vi "多反-镜像-缺陷检测.vi"(4 "底线中心到头部中心偏移量参数":dbl=100.0 format="%#_13g", 5 "头部拟合直径参数":dbl=110.0 format="%#_13g", 7 "胶木铜碎面具偏移_右上0起逆时针":sgl[](array[numeric])=[190.0, 190.0, 190.0, 190.0, 190.0, 190.0, 190.0, 190.0, 190.0, 190.0], 8 "ImgTmps":T8(array[cluster]), 9 "白条面积限度":dbl=200.0 format="%#_13g", 10 "多反调用参数":T9={"IMG_FULL_GRAY_HEAD"=refnum, "IMG_SRC_RO"=refnum, "IMG_Prod_Body_RO"=refnum, "Size_Msk_Half"=0.0, "ROI_Cent"={"Global Rectangle"=[], "Contours"=[]}, "ROI_Prod_Raw"={"Global Rectangle"=[], "Contours"=[]}, "SlotAngles"=[], "img_H_copSlices"=[], "MirroredAngle"=0.0, "SlotCopperParams"={"向外延伸距离"=65.0, "向内延伸距离"=42.0, "排除间隔"=3.0}, "ROIs_Prod_Raw"=[], "MirroredAngles"=[]} {"ROIs_Prod_Raw"."Contours"."Type" items=["No Selection", "Point", "Line", "Rectangle", "Oval", "Polygon", "Freehand Region", "Annulus", "Unused2", "Unused3", "Broken Line", "Freehand Line", "Rotated Rectangle"]; "ROI_Cent"."Contours"."Type" items=["No Selection", "Point", "Line", "Rectangle", "Oval", "Polygon", "Freehand Region", "Annulus", "Unused2", "Unused3", "Broken Line", "Freehand Line", "Rotated Rectangle"]; "ROI_Prod_Raw"."Contours"."Type" items=["No Selection", "Point", "Line", "Rectangle", "Oval", "Polygon", "Freehand Region", "Annulus", "Unused2", "Unused3", "Broken Line", "Freehand Line", "Rotated Rectangle"]}, 11 "镜像编号":i32) -> (0 "ms":cluster{u32, u32, u32}, 1 "头缺量":dbl, 2 "输出簇":T4 {"ROI头缺检测显示"."Contours"."Type" items=["No Selection", "Point", "Line", "Rectangle", "Oval", "Polygon", "Freehand Region", "Annulus", "Unused2", "Unused3", "Broken Line", "Freehand Line", "Rotated Rectangle"]}, 3 "Image Dst Out":T2, 6 "钩外多胶正常":bool)   [LabVIEW 2018]
uses:
  <vilib>/vision/Image Controls.llb/IMAQ Image.ctl
  <vilib>/vision/Measure.llb/Edge Options.ctl
  <vilib>/vision/Measure.llb/Edge Polarity.ctl
  <vilib>/vision/NI_Vision_Development_Module.lvlib
panel:
  in  "原始模板尺寸":T1={"Left"=0, "Top"=0, "Right"=700, "Bottom"=700, "Rotation"=0.0} {"Rotation" format="%.2f"; "Left" scale=0.0..1024.0; "Right" scale=0.0..1024.0}
  out "Image 3":T2(plugin-control)
  out "脏污检测图像":T2(plugin-control)
  out "脏污所处位置信息":dbl[][](array[numeric]) format="%.2f"
  out "脏污数量":i32
  in  "脏污面积下限":T5(array[cluster])=[{"Measurement Parameter"=35, "Range Lower Value"=0.0, "Range Upper Value"=1000.0, "Range"=FALSE, "Measurement Type"=FALSE}] {"Measurement Parameter" items=["Center of Mass X", "Center of Mass Y", "First Pixel X", "First Pixel Y", "Bounding Rect Left", "Bounding Rect Top", "Bounding Rect Right", "Bounding Rect Bottom", "Max Feret Diameter Start X", "Max Feret Diameter Start Y", "Max Feret Diameter End X", "Max Feret Diameter End Y", "Max Horiz. Segment Length Left", "Max Horiz. Segment Length Right", "Max Horiz. Segment Length Row", "-", "Bounding Rect Width", "Bounding Rect Height", "Bounding Rect Diagonal", "Perimeter", "Convex Hull Perimeter", "Holes' Perimeter", "Max Feret Diameter", "Equivalent Ellipse Major Axis", "Equivalent Ellipse Minor Axis", "Equivalent Ellipse Minor Axis (Feret)", "Equivalent Rect Long Side", "Equivalent Rect Short Side", "Equivalent Rect Diagonal", "Equivalent Rect Short Side (Feret)", "Average Horiz. Segment Length", "Average Vert. Segment Length", "Hydraulic Radius", "Waddel Disk Diameter", "-", "Area", "Holes' Area", "Particle & Holes' Area", "Convex Hull Area", "Image Area", "-", "Number of Holes", "Number of Horiz. Segments", "Number of Vert. Segments", "-", "Orientation", "Max Feret Diameter Orientation", "-", "% Area/Image Area", "% Area/(Particle & Holes' Area)", "Ratio of Equivalent Ellipse Axes", "Ratio of Equivalent Rect Sides", "-", "Elongation Factor", "Compactness Factor", "Heywood Circularity Factor", "Type Factor", "-", "Sum X", "Sum Y", "Sum XX", "Sum XY", "Sum YY", "Sum XXX", "Sum XXY", "Sum XYY", "Sum YYY", "-", "Moment of Inertia XX", "Moment of Inertia XY", "Moment of Inertia YY", "Moment of Inertia XXX", "Moment of Inertia XXY", "Moment of Inertia XYY", "Moment of Inertia YYY", "Norm. Moment of Inertia XX", "Norm. Moment of Inertia XY", "Norm. Moment of Inertia YY", "Norm. Moment of Inertia XXX", "Norm. Moment of Inertia XXY", "Norm. Moment of Inertia XYY", "Norm. Moment of Inertia YYY", "Hu Moment 1", "Hu Moment 2", "Hu Moment 3", "Hu Moment 4", "Hu Moment 5", "Hu Moment 6", "Hu Moment 7"]}
  in  "脏污灰度上限":cluster{"Lower value":sgl, "Upper value":sgl}={"Lower value"=2.0, "Upper value"=48.0}
  out "用于打探针查看":T2
  in  "检刀纹_EdgeOptions":T6={"Edge Polarity"=2, "Kernel Size"=3, "Width"=15, "Minimum Edge Strength"=50.0, "Interpolation Type"=enum."Bilinear Fixed", "Data Processing Method"=enum."Average"} {"Edge Polarity" items=["All Edges", "Rising Edges", "Falling Edges"]; "Minimum Edge Strength" format="%.2f"; "Width" step=2; "Kernel Size" step=2}
  out "中心到产品指向角":dbl
  out "Image":T2(plugin-control)
  in  "镜像编号 2":i32
  out "错误输出":errorcluster
  in  "开启调试模式":bool
  in  "开启铜碎调试显示":bool=TRUE
  in  "槽形状参数配置-槽边白条":cluster{"槽形态半长":sgl, "槽形态半宽":sgl}={"槽形态半长"=999.0, "槽形态半宽"=999.0}
  in  "Annulus":T10={"Center X"=0, "Center Y"=0, "Inner Radius"=27, "Outer Radius"=107, "Start Angle"=0.0, "End Angle"=0.0} {"End Angle" min=-90.0 max=90.0 step=1.0 format="%.2f"; "Start Angle" min=-90.0 max=90.0 step=1.0 format="%.2f"; "Center X" scale=0.0..1024.0}
  in  "钩子圆面具偏移":sgl=110.0
  in  "产品高度参考值":sgl=1.0 format="%_3g"
  out "error out 4":errorcluster
  in  "镀锡部分面具偏移_右上0起逆时针":sgl[](array[numeric])=[80.0, 80.0, 80.0, 80.0, 80.0, 80.0, 80.0, 80.0, 80.0, 80.0]
  in  "调整下限消除头部黑区稍亮部位误判作铜碎情况":cluster{"Lower value":i32, "Upper value":i32}={"Lower value"=20, "Upper value"=255}
  in  "头部缺损最大偏差":dbl=2.9999999999999982
  in  "头部边线拟合范围半角":dbl=21.0
  out "error out 6":errorcluster
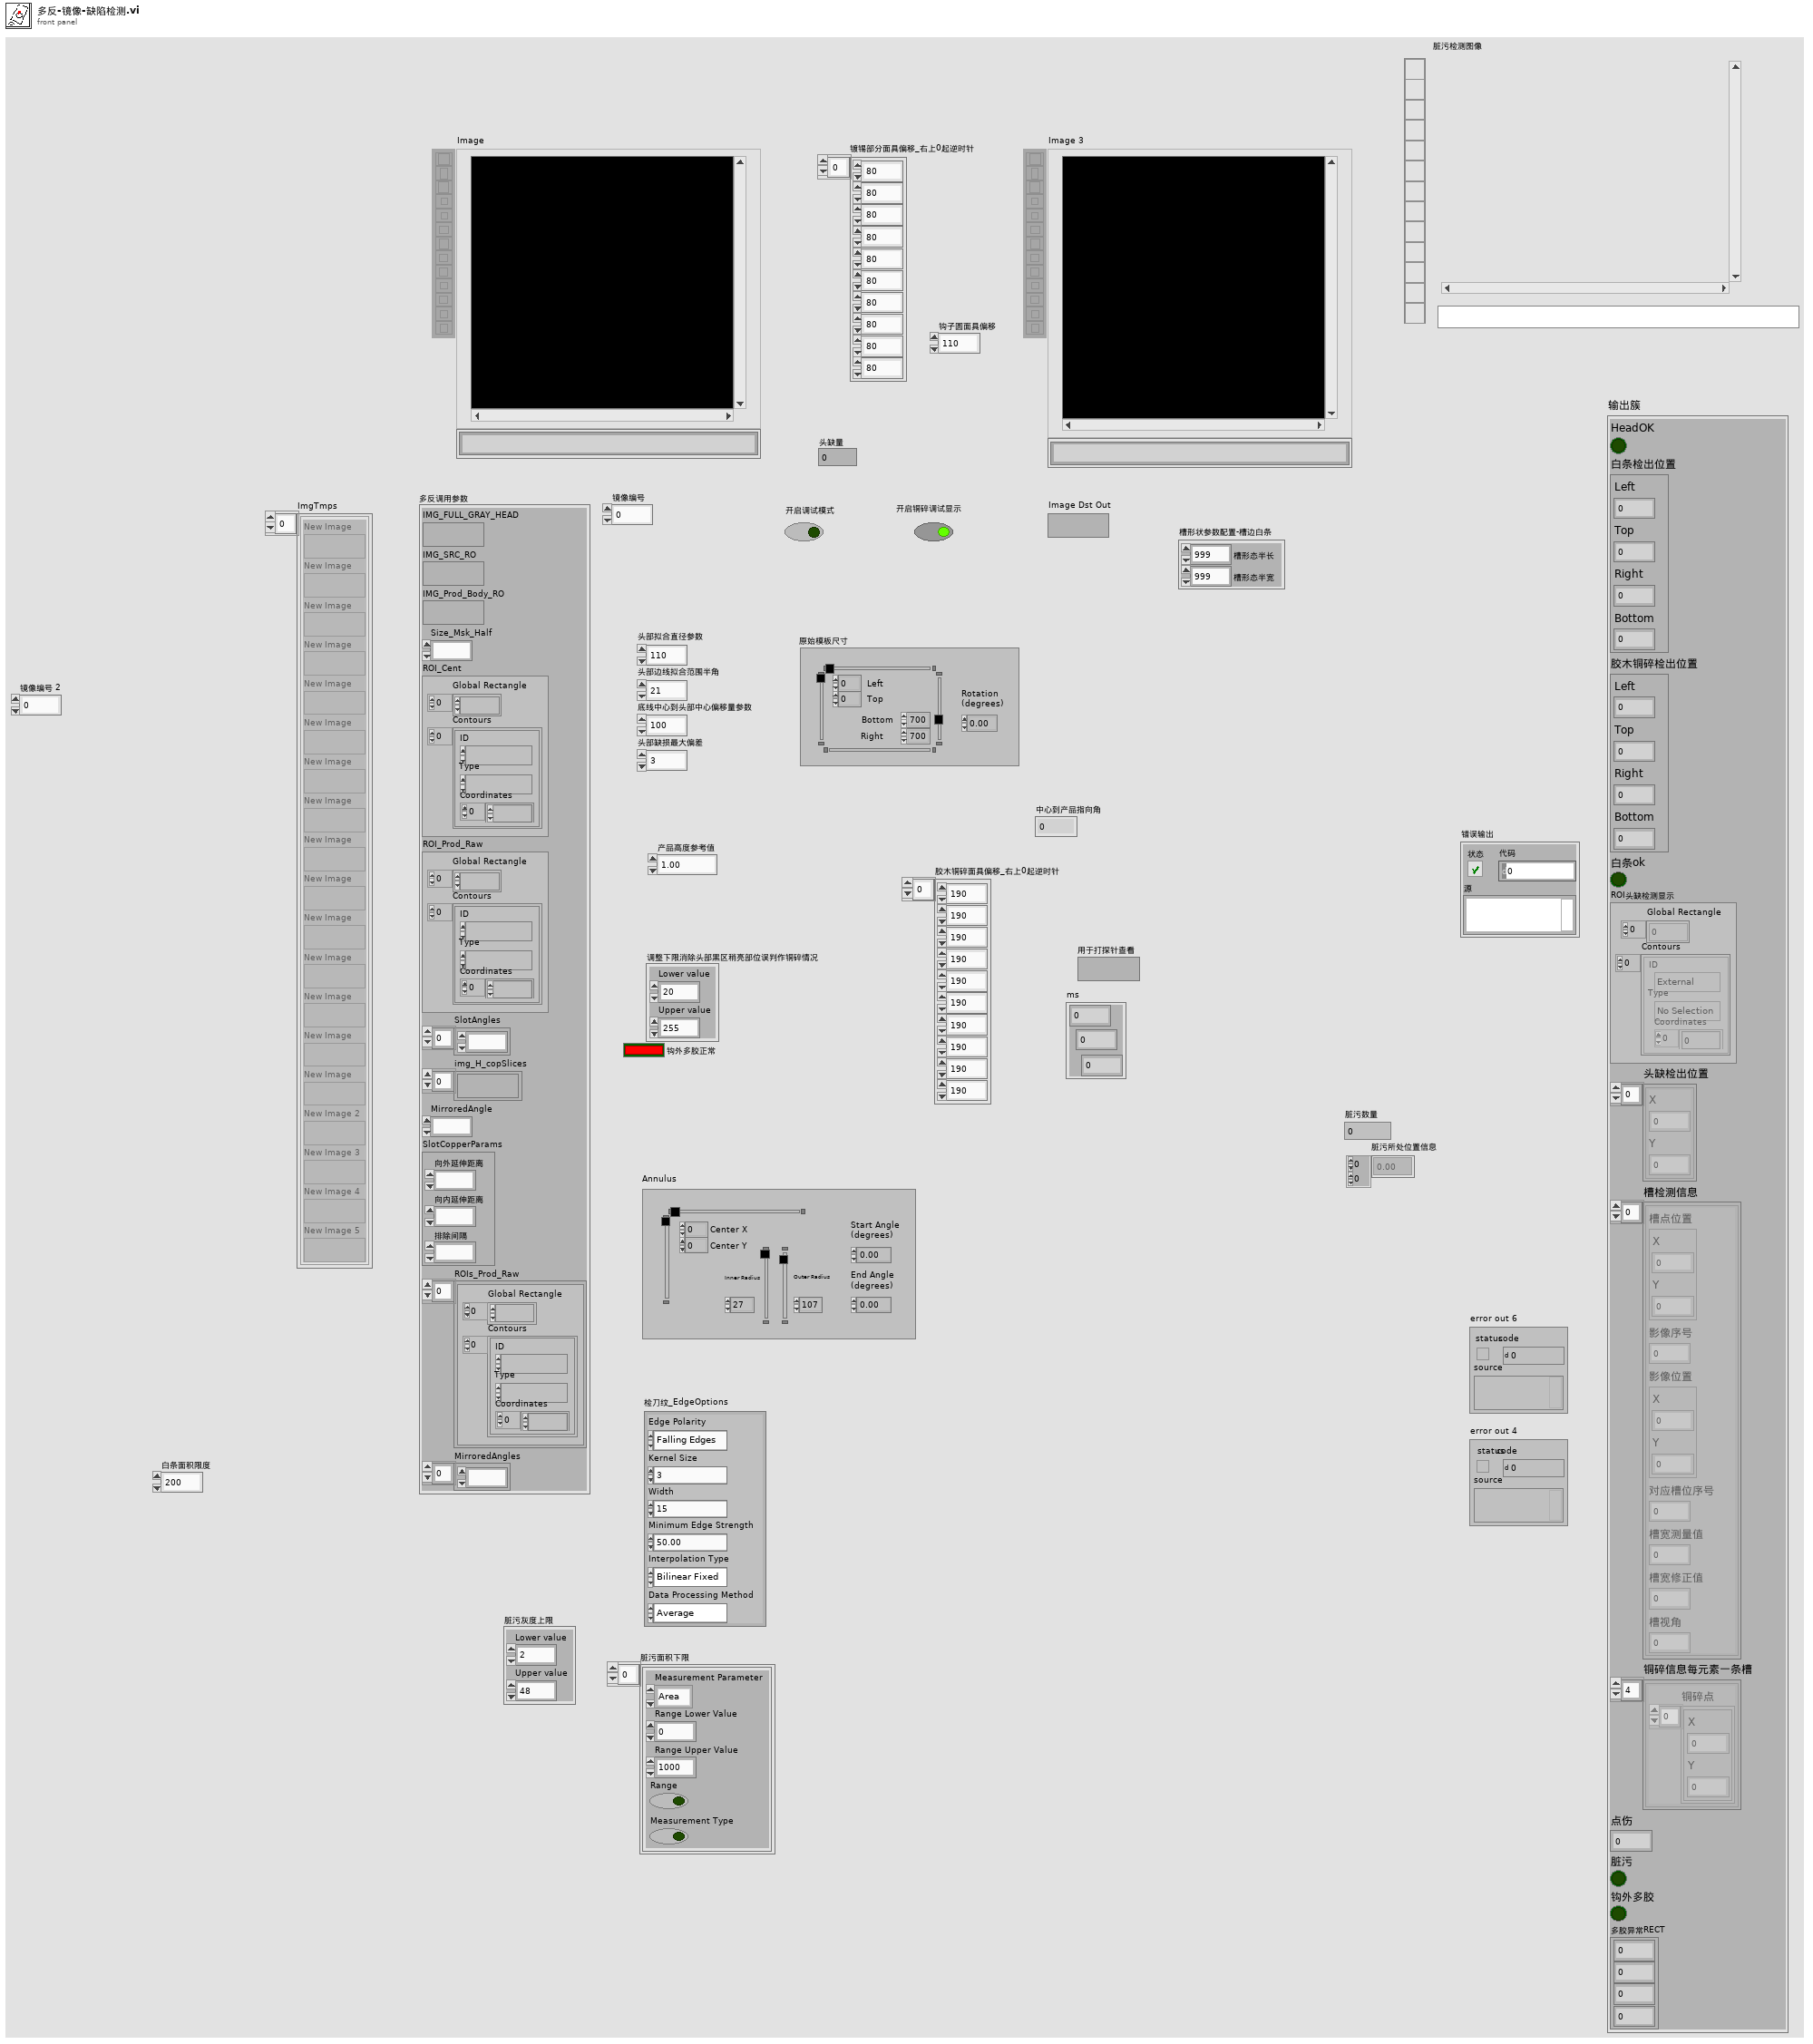
[diagram p1: front panel]
types:
  T1 = typedef "IMAQ Rectangle" = cluster{"Left":i32, "Top":i32, "Right":i32, "Bottom":i32, "Rotation":dbl}
  T2 = typedef "IMAQ Image.ctl" = refnum<image>
  T3 = typedef "ROI Descriptor" = cluster{"Global Rectangle":i32[], "Contours":cluster{"ID":enum32{"External", "Internal"}, "Type":u32, "Coordinates":i32[]}[]}
  T4 = cluster{"HeadOK":bool, "白条检出位置":cluster{"Left":i32, "Top":i32, "Right":i32, "Bottom":i32}, "胶木铜碎检出位置":cluster{"Left":i32, "Top":i32, "Right":i32, "Bottom":i32}, "白条ok":bool, "ROI头缺检测显示":T3, "头缺检出位置":cluster{"X":dbl, "Y":dbl}[], "槽检测信息":cluster{"槽点位置":cluster{"X":sgl, "Y":sgl}, "影像序号":i32, "影像位置":cluster{"X":sgl, "Y":sgl}, "对应槽位序号":i32, "槽宽测量值":dbl, "槽宽修正值":dbl, "槽视角":dbl}[], "铜碎信息每元素一条槽":cluster{"铜碎点":cluster{"X":sgl, "Y":sgl}[]}[], "点伤":dbl, "脏污":bool, "钩外多胶":bool, "多胶异常RECT":cluster{dbl, dbl, dbl, dbl}}
  T5 = cluster{"Measurement Parameter":i32, "Range Lower Value":dbl, "Range Upper Value":dbl, "Range":bool, "Measurement Type":bool}[]
  T6 = typedef "Edge Options.ctl" = cluster{"Edge Polarity":T7, "Kernel Size":u32, "Width":u32, "Minimum Edge Strength":sgl, "Interpolation Type":enum32{"Zero Order", "Bilinear", "Quadratic", "Cubic", "Bilinear Fixed"}, "Data Processing Method":enum32{"Average", "Median"}}
  T7 = typedef "Edge Polarity.ctl" = u32
  T8 = cluster{"New Image":T2, "New Image":T2, "New Image":T2, "New Image":T2, "New Image":T2, "New Image":T2, "New Image":T2, "New Image":T2, "New Image":T2, "New Image":T2, "New Image":T2, "New Image":T2, "New Image":T2, "New Image":T2, "New Image":T2, "New Image 2":T2, "New Image 3":T2, "New Image 4":T2, "New Image 5":T2}[]
  T9 = cluster{"IMG_FULL_GRAY_HEAD":T2, "IMG_SRC_RO":T2, "IMG_Prod_Body_RO":T2, "Size_Msk_Half":dbl, "ROI_Cent":T3, "ROI_Prod_Raw":T3, "SlotAngles":dbl[], "img_H_copSlices":T2[], "MirroredAngle":dbl, "SlotCopperParams":cluster{"向外延伸距离":sgl, "向内延伸距离":sgl, "排除间隔":sgl}, "ROIs_Prod_Raw":T3[], "MirroredAngles":dbl[]}
  T10 = typedef "IMAQ Circle" = cluster{"Center X":i32, "Center Y":i32, "Inner Radius":i32, "Outer Radius":i32, "Start Angle":dbl, "End Angle":dbl}
  T11 = typedef "Image Type" = u32
  T12 = enum32{"AutoM", "Close", "Dilate", "Erode", "Gradient", "Gradient out", "Gradient in", "Hit miss", "Open", "PClose", "POpen", "Thick", "Thin"}
  T13 = enum16{"Get First Edge", "Get First + Last Edge", "Get All Edges", "Get Best Edge"}
  T14 = cluster{"槽点位置":cluster{"X":sgl, "Y":sgl}, "影像序号":i32, "影像位置":cluster{"X":sgl, "Y":sgl}, "对应槽位序号":i32, "槽宽测量值":dbl, "槽宽修正值":dbl, "槽视角":dbl}[]
  T15 = cluster{"New Image":T2, "New Image":T2, "New Image":T2, "New Image":T2, "New Image":T2, "New Image":T2, "New Image":T2, "New Image":T2, "New Image":T2, "New Image":T2, "New Image":T2, "New Image":T2, "New Image":T2, "New Image":T2, "New Image":T2, "New Image 2":T2, "New Image 3":T2, "New Image 4":T2, "New Image 5":T2}
  T16 = cluster{"New Image":T2, "New Image":T2, "New Image":T2, "New Image":T2, "New Image":T2}
  T17 = cluster{"Center (Pixels)":cluster{"X":sgl, "Y":sgl}, "Radius (Pixels)":dbl, "Center (Real-World)":cluster{"X":sgl, "Y":sgl}, "Radius (Real-World)":dbl, "Roundness (Real-World)":dbl, "Average Strength":dbl, "Average SNR (dB)":dbl}
  T18 = typedef "Edge New.ctl" = cluster{"Location (Pixel)":cluster{"X":sgl, "Y":sgl}, "Location (Real-World)":cluster{"X":sgl, "Y":sgl}, "Distance (Pixel)":dbl, "Distance (Real-World)":dbl, "Strength":dbl, "Noise":dbl, "Rising?":bool}
  T19 = cluster{"width":sgl, "point":cluster{"X":sgl, "Y":sgl}}[]
  T20 = cluster{"槽点位":cluster{"X":sgl, "Y":sgl}, "产品位":cluster{"X":sgl, "Y":sgl}, "各槽角":dbl[], "中心位":cluster{"X":sgl, "Y":sgl}, "中心产品半径":sgl, "最接近槽角序号":i32, "槽在中心到产品连线所在侧":enum16{"左侧-逆时针向", "右侧-顺时针向"}, "中心位到产品位指向角":sgl}
  T21 = cluster{"产品位":cluster{"X":sgl, "Y":sgl}, "槽点位":cluster{"X":sgl, "Y":sgl}, "产品位指向角度":sgl, "产品底线半径":sgl, "向外延伸距离":sgl, "向内延伸距离":sgl, "排除间隔":sgl}
  T22 = cluster{"槽点位置":cluster{"X":sgl, "Y":sgl}, "影像序号":i32, "影像位置":cluster{"X":sgl, "Y":sgl}, "对应槽位序号":i32, "槽宽测量值":dbl, "槽宽修正值":dbl, "槽视角":dbl}
  T23 = cluster{"ImageCut":T2, "ImageCutGray":T2, "ImageMask":T2, "ImageInter1":T2, "ImageInter2":T2, "ImageInter3":T2}
  T24 = cluster{"Left":i32, "Top":i32, "Right":i32, "Bottom":i32}
  T25 = cluster{"y":dbl, dbl, dbl, dbl, "MirroredAngle":dbl}
  T26 = typedef "Search Line.ctl" = cluster{"Start Point":cluster{"X":sgl, "Y":sgl}, "End Point":cluster{"X":sgl, "Y":sgl}, "Edge Info":T18[], "Edge Map":dbl[], "Calibration Valid":bool}
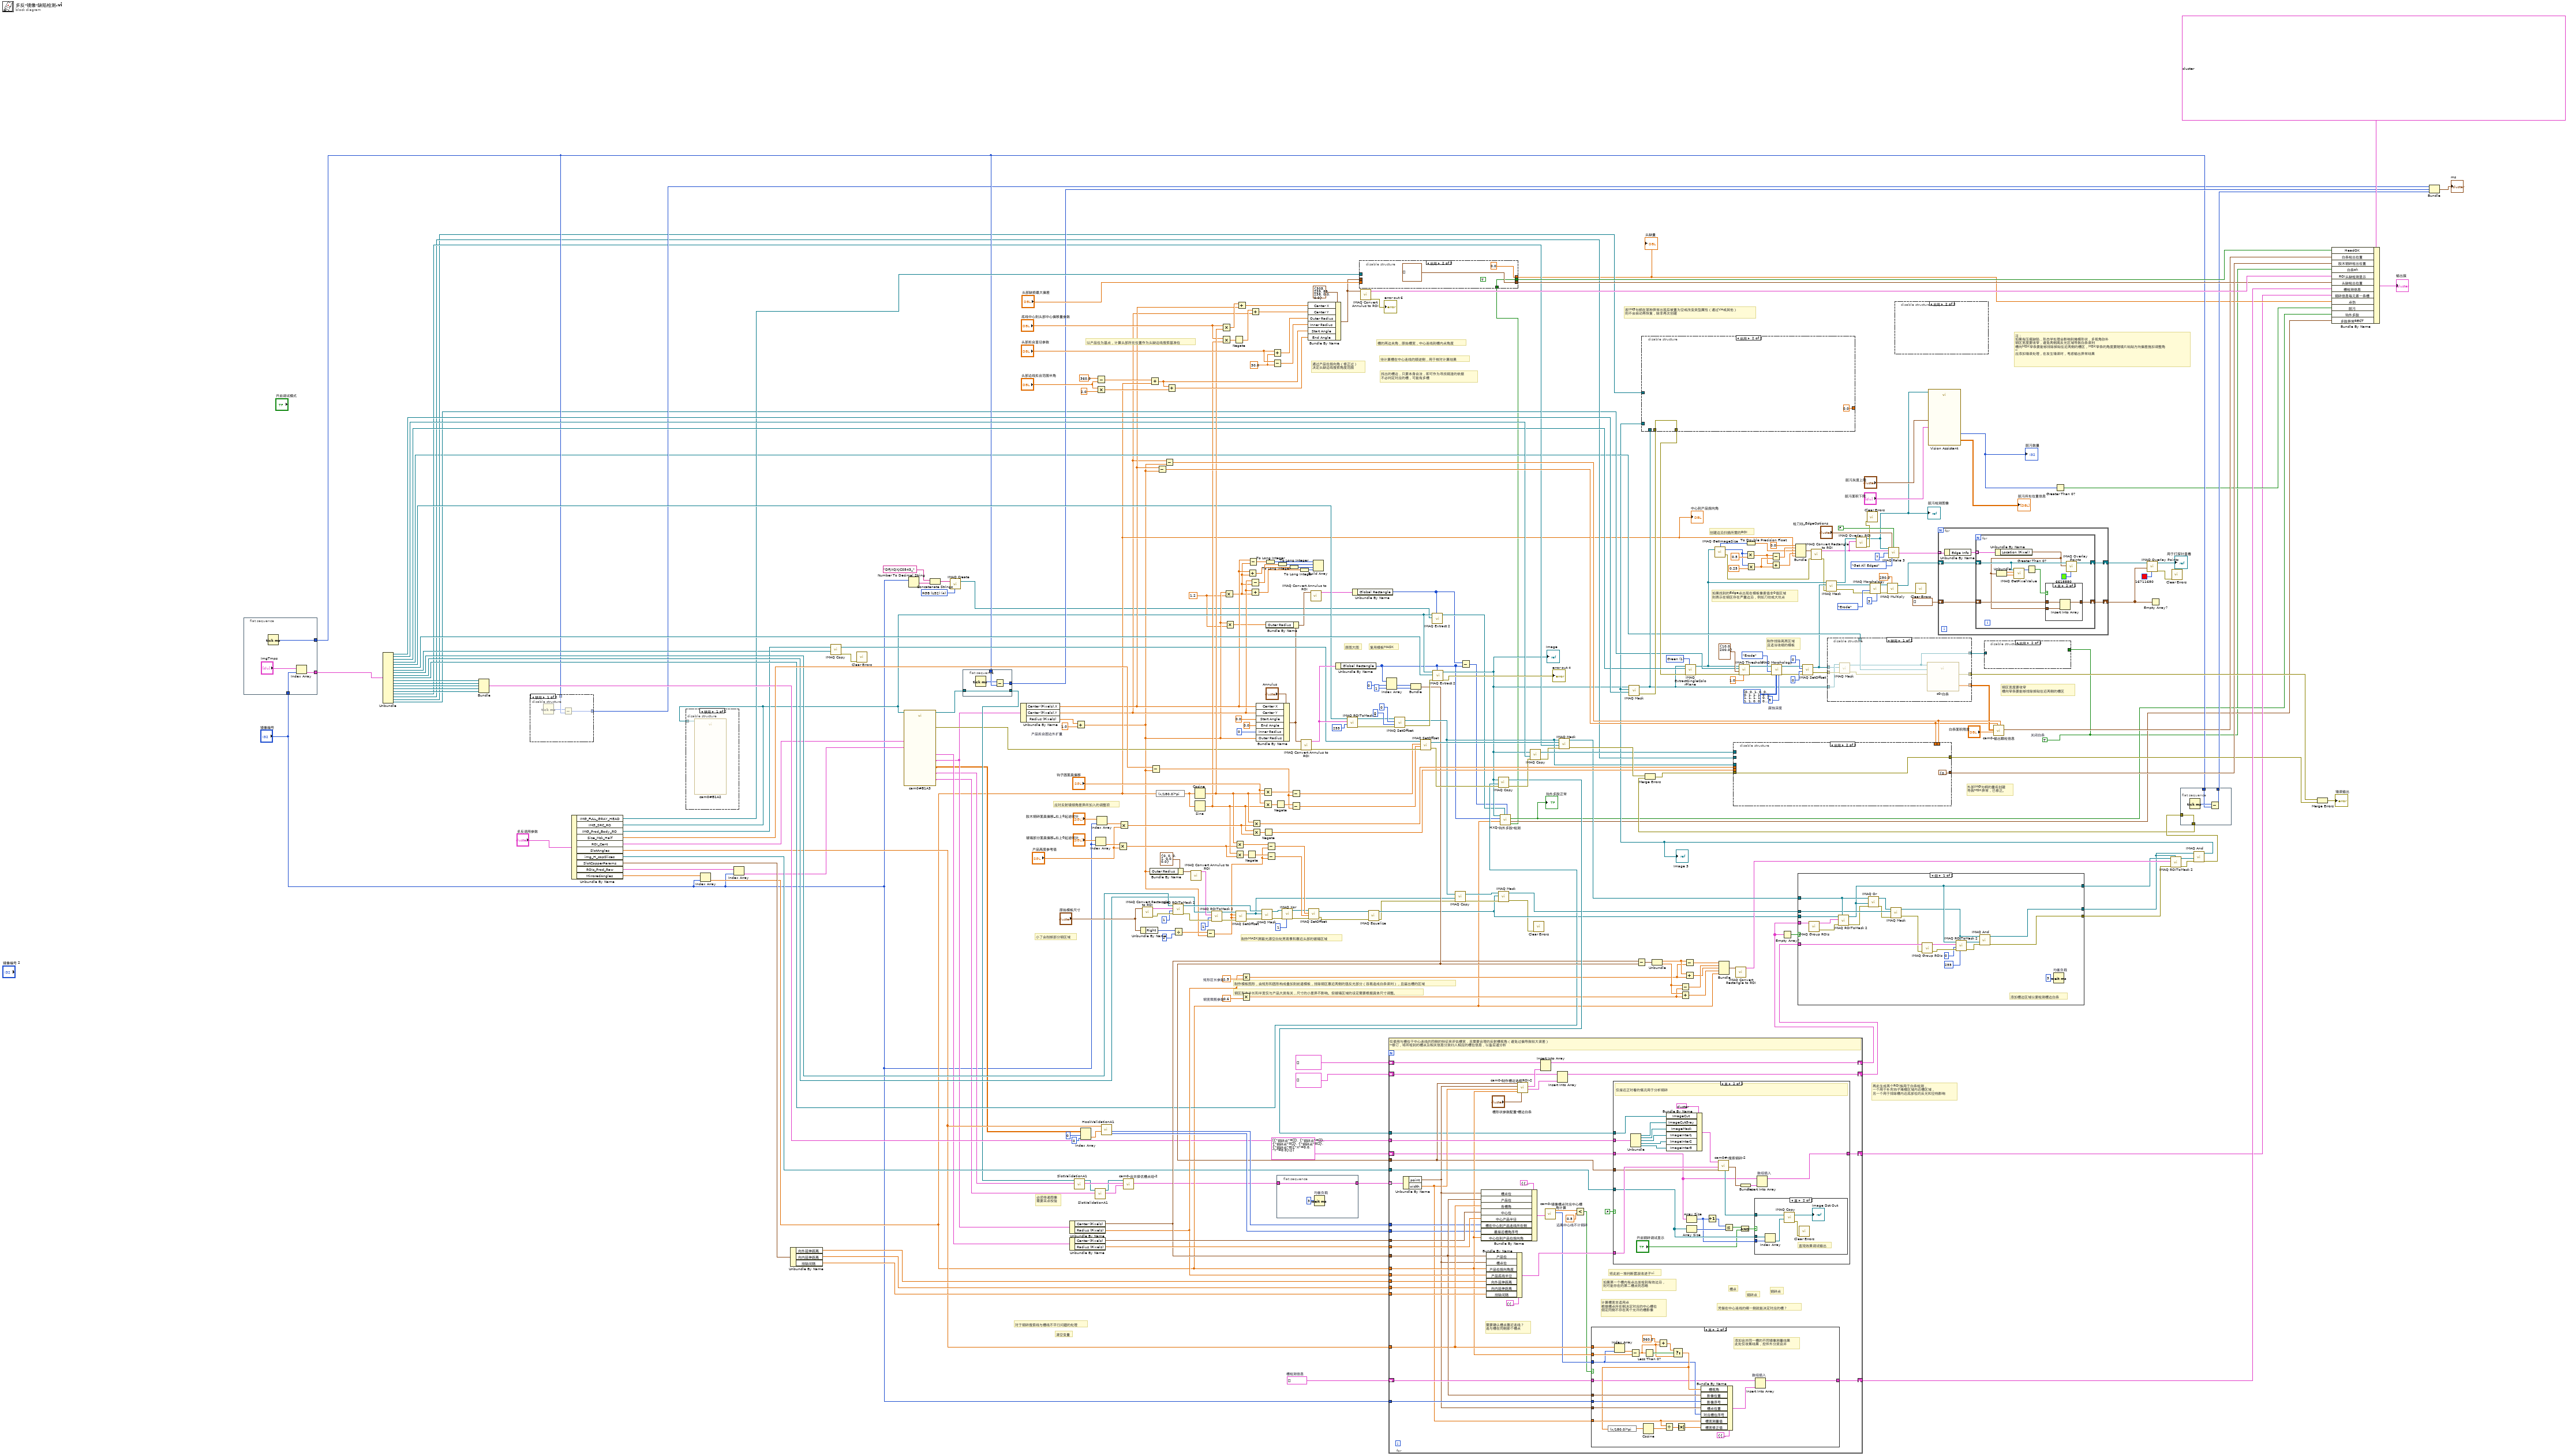
[diagram p0: block diagram]
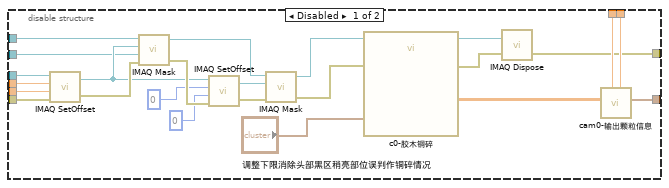
[diagram p3: hidden frame]
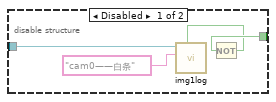
[diagram p4: hidden frame]
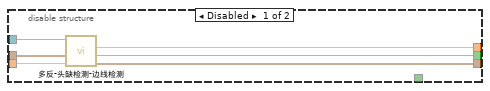
[diagram p6: hidden frame]
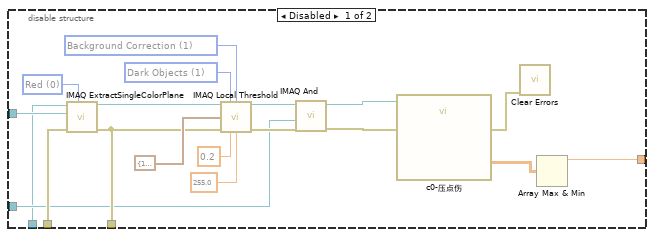
[diagram p7: hidden frame]
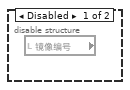
[diagram p8: hidden frame]
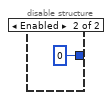
[diagram p10: hidden frame]
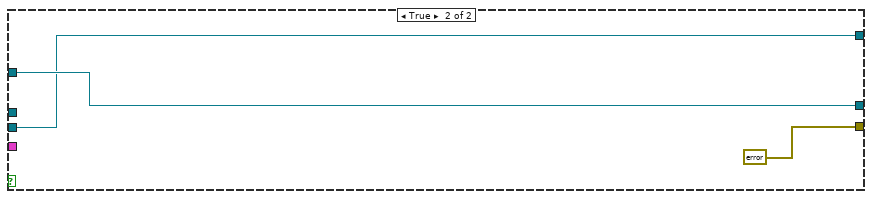
[diagram p11: hidden frame]
diagram:
  w1 = TRUE  # 关闭白条
  w26 = T11 4 items=["Grayscale (U8)", "Grayscale (I16)", "Grayscale (SGL)", "Complex (CSG)", "RGB (U32)", "HSL (U32)", "RGB (U64)", "Grayscale (U16)"] ("Image Type")
  w12 = 1.2 ("y")
  w120 = 1.0  # 产品拟合圆边外扩量
  w150 = T14 []  # 槽检测信息
  w181 = 30.0 ("y")
  w190 = 1.5  # 矩形区长参数
  w189 = 0.6  # 铜宽裁剪参数
  w280 = 5  # 腐蚀深度
  w292 = 1 items=["Red", "Green", "Blue", "Hue", "Saturation", "Luminance", "Value", "Intensity"] ("Color Plane")
  # "如果找到的Edge点出现在模板像素值非0值区域\n则表示在铜区存在严重边沿，例如刀纹或大坑点"
  # "创建边沿扫描所需的ROI"
  # "铜区宽度要收窄\n槽向窄条要能够排除掉贴住近两侧的槽区"
  # "注：\n如果有压痕缺陷，形态学处理会影响到掩模形状，多视角弥补\n铜区宽度要收窄，避免两侧高反光区域导致白条误判\n槽向MSK窄条要能够排除掉贴住近两侧的槽区，MSK窄条的角度要随镜片粘贴方向偏差施加调整角\n--\n应添加错误处理，在发生错误时，考虑输出异常结果"
  # "若IMG句柄在某种异常出现后被置为空或改变类型属性（通过VA或其他）\n则不会自动再恢复，除非再次创建"
  # "外部IMG句柄的重名创建\n导致MSK异常，已修正。"
  # "再此生成两个ROI族用于白条检测，\n一个用于补充钩子掩模区域内近槽区域，\n另一个用于排除槽内近底部位的反光和空档影响"
  # "通过产品位指向角（修正过）\n决定头缺边线搜索角度范围"
  # "以产品位为基点，计算头部所在位置作为头缺边线搜索基准位"
  # "小了会削掉部分铜区域"
  # "应对反射镜倾角差异所加入的调整项"
  # "铜区形态半长和半宽仅与产品大类有关，尺寸的小差异不影响。但镀锡区域的设定需要根据具体尺寸调整。"
  # "制作模板图形，由矩形和圆形构成叠加到前道模板，排除铜区靠近两侧的强反光部分（容易造成白条误判），且留出槽的区域"
  # "制作MASK屏蔽光源空白处亮背景和靠近头部的镀锡区域"
  # "制作排除高亮区域\n且适当收缩的模板"
  # "对于铜碎搜索线与槽线不平行问题的处理"
  # "清空变量"
  # "必须传递图像\n需要采点校验"
  # "复用模板MASK"
  # "原图大图"
  # "找出的槽边，只要本身合法，即可作为寻找铜渣的依据\n不必判定对应的槽，可能有多槽"
  # "待计算槽在中心连线的顺逆侧，用于核对计算结果"
  # "槽的两边夹角，原始槽宽，中心连线到槽内点角度"
  n1 = flat-sequence {
    tunnel: "镜像编号" -> [w316]
    tunnel: [w315] -> w115
    tunnel: [w314] -> w108
    frame #0 {
      n2 = Tick Count (ms)() -> (millisecond timer value=w315:u32)
      n3 = Index Array(array="ImgTmps", index=w316) -> (element=w314:T15)
    }
  }
  n4 = Unbundle(w108) -> ("New Image"=w144:T2, "New Image"=w143:T2, "New Image"=w138:T2, "New Image"=w93:T2, "New Image"=w139:T2, "New Image"=w140:T2, "New Image"=w128:T2, "New Image"=w142:T2, "New Image"=w141:T2, "New Image"=w137:T2, "New Image"=w109:T2, "New Image"=w110:T2, "New Image"=w111:T2, "New Image"=w112:T2, "New Image"=w113:T2, "New Image 2"=w105:T2, "New Image 3"=w104:T2, "New Image 4"=w103:T2, "New Image 5"=w94:T2)
  n5 = Bundle("New Image"=w109, "New Image"=w110, "New Image"=w111, "New Image"=w112, "New Image"=w113) -> (w136:T16)  [unwired: 1 in]
  n6 = disable-structure shown="禁用" {
    disable-tunnel: w115 -> [w319 _]
    disable-tunnel: [w318 u32 0] -> w114
    frame Disabled {
      n7 = Tick Count (ms)() -> (millisecond timer value=w317:u32)
      n8 = Subtract(x=w317, y=w319) -> (x-y=w318:u32)
    }
    frame Enabled {
    }
  }
  n9 = Unbundle By Name("多反调用参数") -> ("IMG_FULL_GRAY_HEAD"=w135:T2, "IMG_SRC_RO"=w31:T2, "IMG_Prod_Body_RO"=w129:T2, "Size_Msk_Half"=w159:dbl, "ROI_Cent"=w53:T3, "SlotAngles"=w133:dbl[], "img_H_copSlices"=w158:T2[], "SlotCopperParams"=w157:cluster{"向外延伸距离":sgl, "向内延伸距离":sgl, "排除间隔":sgl}, "ROIs_Prod_Raw"=w132:T3[], "MirroredAngles"=w131:dbl[])
  n10 = disable-structure shown="禁用" {
    disable-tunnel: w31 -> [w321 _]
    frame Disabled {
      n11 = call "cam0#B1A2"("Image In"=w321) -> ()  [unwired: 20 in, 7 out]
    }
    frame Enabled {
    }
  }
  n12 = Index Array(array=w131, index="镜像编号") -> (element=w37:dbl)
  "中心到产品指向角" <- w37
  n13 = Index Array(array=w132, index="镜像编号") -> (element=w52:T3)
  n14 = Unbundle By Name(w157) -> ("向外延伸距离"=w156:sgl, "向内延伸距离"=w155:sgl, "排除间隔"=w154:sgl)
  n15 = call "IMAQ Copy"("Image Dst"=w128, "Image Src"=w129) -> ("error out"=w98:errorcluster, "Image Dst Out"=w134:T2)  [unwired: 4 in]
  n16 = call <vilib>:"Clear Errors.vi"("error in (no error)"=w98) -> ()  [unwired: 5 in, 2 out]
  n17 = call "cam0#B1A3"("Image In"=w31, "ROI Descriptor (Cent)"=w53, "ROI Descriptor (cir_pro_raw)"=w52) -> ("Caliper Results (angle_Cent_pro_fine)"=w49:sgl[][], "Image Out"=w55:T2, "Fitted Circle (Cent)"=w51:T17, "Fitted Circle (cir_pro_Fine)"=w50:T17, "Edge Information (edge_Find_SlotSidesLo)"=w48:T18[], "Edge Information (edge_Find_SlotSidesHi)"=w47:T18[], "error out"=w54:errorcluster)  [unwired: 18 in]
  n18 = Number To Decimal String(number="镜像编号") -> (decimal integer string=w29:string)  [unwired: 1 in]
  n19 = Concatenate Strings("DFJXQXJC0543_" ("字符串"), w29) -> (w28:string)
  n20 = call "IMAQ Create"("Image Name"=w28, "Image Type"=w26) -> ("New Image"=w8:T2)  [unwired: 3 in, 1 out]
  n21 = flat-sequence {
    tunnel: [w325] -> w124
    tunnel: w115 -> [w324]
    tunnel: [w322] -> w119
    tunnel: w55 -> [w322]
    frame #0 {
      n22 = Tick Count (ms)() -> (millisecond timer value=w323:u32)
      n23 = Subtract(x=w323, y=w324) -> (x-y=w325:u32)
    }
  }
  n24 = Unbundle By Name(w50) -> ("Center (Pixels).X"=w34:sgl, "Center (Pixels).Y"=w33:sgl, "Radius (Pixels)"=w121:dbl)
  n25 = Unbundle By Name(w50) -> ("Center (Pixels)"=w192:cluster{"X":sgl, "Y":sgl}, "Radius (Pixels)"=w191:dbl)
  n26 = Unbundle By Name(w51) -> ("Center (Pixels)"=w310:cluster{"X":sgl, "Y":sgl}, "Radius (Pixels)"=w276:dbl)
  n27 = call "SlotValidationA1.vi"("EdgeSlotSides"=w48, "ImageIn"=w119) -> ("槽点"=w278:T19, "ImageOut"=w277:T2)  [unwired: 8 in]
  n28 = Add(x=w121, y=w120) -> (x+y=w13:dbl)
  n29 = Index Array ("从反射镜内产品到中心产品连线角度")(array=w49, index (row)=0 ("禁用的索引 (行)"), index (col)=0 ("禁用的索引 (列)")) -> (element=w308:sgl)
  n30 = call "SlotValidationA1.vi"("EdgeSlotSides"=w47, "ImageIn"=w277) -> ("槽点"=w279:T19, "ImageOut"=w147:T2)  [unwired: 8 in]
  n31 = Index Array(array="镀锡部分面具偏移_右上0起逆时针", index="镜像编号") -> (element=w254:sgl)
  n32 = Subtract(x=360.0, y="头部边线拟合范围半角") -> (x-y=w177:dbl)
  n33 = Multiply(x="头部边线拟合范围半角", y=2.0) -> (x*y=w174:dbl)
  n34 = Index Array(array="胶木铜碎面具偏移_右上0起逆时针", index="镜像编号") -> (element=w268:sgl)
  n35 = call "HookValidationA1.vi"("中心到镜像产品连线角度"=w308, "各槽角"=w133) -> ("槽角序号"=w275:i32, "槽在中心到产品连线所在侧"=w309:enum16{"左侧-逆时针向", "右侧-顺时针向"})  [unwired: 7 in, 1 out]
  n36 = Multiply(x=w254, y="产品高度参考值") -> (x*y=w250:sgl)
  n37 = Multiply(x=w268, y="产品高度参考值") -> (x*y=w267:sgl)
  n38 = call "cam0-合并择优槽点组-2.vi"("槽点组优先"=w279, "槽点组初步"=w278, "ImageIn"=w147) -> ("槽点组合并"=w3:T19)  [unwired: 7 in, 1 out]
  n39 = Unbundle By Name("原始模板尺寸") -> ("Right"=w248:i32)
  n40 = call "IMAQ Convert Rectangle to ROI"("Rectangle"="原始模板尺寸") -> ("error out"=w242:errorcluster, "ROI Descriptor"=w240:T3)  [unwired: 8 in]
  n41 = Add(x=w177, y=w37) -> (x+y=w173:dbl)
  n42 = Bundle By Name(cluster=T10 {"Center X"=0, "Center Y"=0, "Inner Radius"=0, "Outer Radius"=1, "Start Angle"=0.0, "End Angle"=0.0} ("Annulus"), "Outer Radius"=w13) -> (w238:T10)
  n43 = Subtract(x=w159, y=w13) -> (x-y=w297:dbl)
  n44 = expression code="(x/180.0)*pi" ("degrees to radians")(w37) -> (w303:dbl)
  n45 = Subtract(x=w34, y=w13) -> (x-y=w185:dbl)
  n46 = Subtract(x=w33, y=w13) -> (x-y=w257:dbl)
  n47 = Add(x=w173, y=w174) -> (x+y=w172:dbl)
  n48 = call "IMAQ ROIToMask 2"("error in (no error)"=w242, "Filling Value (255)"=1, "ROI Descriptor"=w240, "Image"=w142) -> ("error out"=w241:errorcluster, "Image Out"=w245:T2)  [unwired: 5 in, 1 out]
  n49 = Divide(x=w248, y=2) -> (x/y=w239:dbl)
  n50 = call "IMAQ Convert Annulus to ROI"("Annulus"=w238) -> ("ROI Descriptor"=w235:T3)  [unwired: 8 in, 1 out]
  n51 = Cosine(x=w303) -> (cos(x)=w169:dbl)
  n52 = Sine(x=w303) -> (sin(x)=w166:dbl)
  n53 = Subtract(x=w239, y=w13) -> (x-y=w232:dbl)
  n54 = call "IMAQ ROIToMask 2"("error in (no error)"=w241, "Filling Value (255)"=1, "ROI Descriptor"=w235, "Image"=w141) -> ("error out"=w244:errorcluster, "Image Out"=w243:T2)  [unwired: 5 in, 1 out]
  n55 = Multiply(x="底线中心到头部中心偏移量参数", y=w169) -> (x*y=w168:dbl)
  n56 = Multiply(x="底线中心到头部中心偏移量参数", y=w166) -> (x*y=w165:dbl)
  n57 = Multiply(x=w13, y=w12) -> (x*y=w32:dbl)
  n58 = Multiply(x=w13, y=w12) -> (x*y=w14:dbl)
  n59 = Negate(x=w165) -> (-x=w164:dbl)
  n60 = Multiply(x=w169, y=w250) -> (x*y=w234:dbl)
  n61 = Multiply(x=w166, y=w250) -> (x*y=w251:dbl)
  n62 = call "IMAQ SetOffset"("error in (no error)"=w244, "Y Offset"=w232, "X Offset"=w232, "Image"=w243) -> ("error out"=w246:errorcluster, "Image Out"=w186:T2)
  n63 = Add(x=w168, y=w34) -> (x+y=w171:dbl)
  n64 = Multiply(x=w191, y=w190) -> (x*y=w188:dbl)
  n65 = Multiply(x=w191, y=w189) -> (x*y=w187:dbl)
  n66 = Negate(x=w251) -> (-x=w233:dbl)
  n67 = Add(x=w34, y=w32) -> (x+y=w20:dbl)
  n68 = Subtract(x=w34, y=w32) -> (x-y=w24:dbl)
  n69 = Subtract(x=w33, y=w32) -> (x-y=w22:dbl)
  n70 = Add(x=w33, y=w32) -> (x+y=w18:dbl)
  n71 = Add(x=w164, y=w33) -> (x+y=w170:dbl)
  n72 = Multiply(x=w169, y=w267) -> (x*y=w270:dbl)
  n73 = Multiply(x=w166, y=w267) -> (x*y=w272:dbl)
  n74 = Bundle By Name(cluster="Annulus", "Center X"=w34, "Center Y"=w33, "Start Angle"=0.0, "End Angle"=0.0, "Inner Radius"=0, "Outer Radius"=w13) -> (w15:T10)
  n75 = call "IMAQ Mask"("error in (no error)"=w246, "Image Mask"=w186, "Image Src"=w245) -> ("error out"=w219:errorcluster, "Image Dst Out"=w225:T2)  [unwired: 2 in]
  n76 = Multiply(x="钩子圆面具偏移", y=w169) -> (x*y=w300:dbl)
  n77 = Multiply(x="钩子圆面具偏移", y=w166) -> (x*y=w301:dbl)
  n78 = Negate(x=w272) -> (-x=w271:dbl)
  n79 = To Long Integer(number=w24) -> (32bit integer=w23:i32)
  n80 = Bundle By Name(cluster=w15, "Outer Radius"=w14) -> (w11:T10)
  n81 = Subtract(x=w234, y=w232) -> (x-y=w231:dbl)
  n82 = Subtract(x=w233, y=w232) -> (x-y=w230:dbl)
  n83 = Add(x="头部拟合直径参数", y=w181) -> (x+y=w180:dbl)
  n84 = Subtract(x="头部拟合直径参数", y=w181) -> (x-y=w179:dbl)
  n85 = Negate(x=w301) -> (-x=w299:dbl)
  n86 = flat-sequence {
    tunnel: w3 -> [w327]
    tunnel: [w327] -> w2
    frame #0 {
      n87 = Wait (ms) "均衡负载"(milliseconds to wait=u32 3 ("等待时间（毫秒）")) -> ()  [unwired: 1 out]
    }
  }
  n88 = To Long Integer(number=w22) -> (32bit integer=w21:i32)
  n89 = call "IMAQ Xor"("Constant"=i64 1, "error in (no error)"=w219, "Image Src A"=w225) -> ("error out"=w218:errorcluster, "Image Dst Out"=w224:T2)  [unwired: 7 in]
  n90 = To Long Integer(number=w20) -> (32bit integer=w19:i32)
  n91 = Subtract(x=w300, y=w297) -> (x-y=w265:dbl)
  n92 = Subtract(x=w299, y=w297) -> (x-y=w266:dbl)
  n93 = To Long Integer(number=w18) -> (32bit integer=w17:i32)
  n94 = call "IMAQ Convert Annulus to ROI"("error in (no error)"=w54, "Annulus"=w15) -> ("error out"=w304:errorcluster, "ROI Descriptor"=w294:T3)  [unwired: 7 in]
  n95 = Bundle By Name(cluster=T10 {"Center X"=305, "Center Y"=239, "Inner Radius"=89, "Outer Radius"=238, "Start Angle"=0.0, "End Angle"=0.0} ("Annulus"), "Center X"=w171, "Center Y"=w170, "Outer Radius"=w180, "Inner Radius"=w179, "Start Angle"=w173, "End Angle"=w172) -> (w163:T10)
  n96 = call "IMAQ SetOffset"("error in (no error)"=w218, "Y Offset"=w230, "X Offset"=w231, "Image"=w224) -> ("error out"=w96:errorcluster, "Image Out"=w107:T2)
  n97 = call "IMAQ Convert Annulus to ROI"("Annulus"=w11) -> ("ROI Descriptor"=w10:T3)  [unwired: 8 in, 1 out]
  n98 = Build Array(w23, w21, w19, w17) -> ()  [unwired: 1 out]
  n99 = Unbundle By Name(w294) -> ("Global Rectangle"=w7:i32[])
  n100 = call "IMAQ ROIToMask 2"("Filling Value (255)"=255, "ROI Descriptor"=w294, "Image"=w139) -> ("error out"=w213:errorcluster, "Image Out"=w214:T2)  [unwired: 6 in, 1 out]
  n101 = Unbundle By Name(w10) -> ("Global Rectangle"=w9:i32[])
  n102 = call "IMAQ Convert Annulus to ROI"("Annulus"=w163) -> ("error out"=→"error out 6":errorcluster, "ROI Descriptor"=w149:T3)  [unwired: 8 in]
  n103 = call "IMAQ Equalize"("error in (no error)"=w96, "Image Src"=w107) -> ("error out"=w95:errorcluster, "Image Dst Out"=w106:T2)  [unwired: 8 in]
  n104 = Index Array(array=w7, index #1=0 ("索引"), index #2=1 ("索引")) -> (element #1=w261:i32, element #2=w260:i32)
  n105 = call "IMAQ SetOffset"("error in (no error)"=w213, "Y Offset"=0, "X Offset"=0, "Image"=w214) -> ("error out"=w216:errorcluster, "Image Out"=w211:T2)
  n106 = Bundle(w261, w260) -> (w203:cluster{i32, i32})  [unwired: 1 in]
  n107 = call "IMAQ SetOffset"("error in (no error)"=w304, "Y Offset"=w266, "X Offset"=w265, "Image"=w134) -> ("error out"=w259:errorcluster, "Image Out"=w215:T2)
  n108 = call "IMAQ Extract 2"("Optional Rectangle"=w9, "Image Dst"=w8, "Image Src"=w31) -> ("Image Dst Out"=w25:T2)  [unwired: 7 in, 1 out]
  n109 = call "IMAQ Extract 2"("Optional Rectangle"=w7, "error in (no error)"=w216, "Image Dst"=w140, "Image Src"=w31) -> ("error out"=→"error out 4":errorcluster, "Image Dst Out"=w36:T2)  [unwired: 6 in]
  "Image" <- w36
  n110 = call "IMAQ Copy"("error in (no error)"=w95, "Image Dst"=w186, "Image Src"=w211) -> ("error out"=w209:errorcluster, "Image Dst Out"=w229:T2)  [unwired: 3 in]
  n111 = Subtract(x=w9, y=w7) -> (x-y=w16:i32[])
  n112 = call "IMAQ Copy"("error in (no error)"=w259, "Image Dst"=w137, "Image Src"=w36) -> ("error out"=w264:errorcluster, "Image Dst Out"=w220:T2)  [unwired: 3 in]
  n113 = for {
    tunnel: w2 -> [w366] mode=indexing
    tunnel: w310 -> [w353]
    tunnel: w309 -> [w341]
    tunnel: w192 -> [w355]
    tunnel: w37 -> [w345]
    tunnel: w191 -> [w364]
    tunnel: w156 -> [w363]
    tunnel: w155 -> [w362]
    tunnel: w154 -> [w361]
    shift-right: [w360] -> w146
    shift-left: w150 -> [w359]
    tunnel: "镜像编号" -> [w349]
    tunnel: w133 -> [w354]
    tunnel: w276 -> [w352]
    tunnel: w275 -> [w340]
    tunnel: w203 -> [w338]
    tunnel: w220 -> [w332]
    tunnel: w158 -> [w348]
    tunnel: w136 -> [w347]
    shift-right: [w343] -> w222
    shift-left: T3[] [] ("ROI Descriptors") -> [w344]
    shift-right: [w334] -> w160
    shift-left: T3[] [] ("ROI Descriptors") -> [w335]
    shift-right: [w330] -> w60
    shift-left: cluster{"铜碎点":cluster{"X":sgl, "Y":sgl}[]}[] [{"铜碎点"=[]}, {"铜碎点"=[]}, {"铜碎点"=[]}, {"铜碎点"=[]}, {"铜碎点"=[{"X"=0.0, "Y"=0.0}]}] ("铜碎信息每元素一条槽") -> [w331]
    w350 = 0.5  # 远离中心线不计铜碎
    # "计算槽宽非适用点\n根据槽点所在侧决定对应的中心槽位\n假定同侧不存在两个允许的槽影像"
    # "铜碎点"
    # "铜碎点"
    # "槽点"
    # "凭借在中心连线的哪一侧就能决定对应的槽？"
    # "将此前一堆判断套装收进子vi"
    # "如果第一个槽内有点出发检到有效边沿，\n则可能存在的第二槽点则忽略"
    # "需要确认槽点靠近连线？\n选与槽在同侧那个槽点"
    # "仅使用与槽位于中心连线的同侧的特征来评估槽宽，且需要合理的反射槽视角（避免过偏导致较大误差）\n--修订，将所检到的槽点及相关信息分类归入相应的槽位信息，以备后道分析"
    n114 = Unbundle By Name(w366) -> ("point"=w337:cluster{"X":sgl, "Y":sgl}, "width"=w336:sgl)
    n115 = Bundle By Name(cluster=T20 {"槽点位"={"X"=125.0, "Y"=75.0}, "产品位"={"X"=150.0, "Y"=100.0}, "各槽角"=[], "中心位"={"X"=100.0, "Y"=100.0}, "中心产品半径"=0.0, "最接近槽角序号"=0, "槽在中心到产品连线所在侧"=enum."左侧-逆时针向", "中心位到产品位指向角"=0.0} ("位置参数"), "槽点位"=w337, "产品位"=w355, "各槽角"=w354, "中心位"=w353, "中心产品半径"=w352, "槽在中心到产品连线所在侧"=w341, "最接近槽角序号"=w340, "中心位到产品位指向角"=w345) -> (w356:T20)
    n116 = Bundle By Name(cluster=T21 {"产品位"={"X"=0.0, "Y"=0.0}, "槽点位"={"X"=0.0, "Y"=0.0}, "产品位指向角度"=0.0, "产品底线半径"=0.0, "向外延伸距离"=0.0, "向内延伸距离"=0.0, "排除间隔"=0.0} ("输入参数信息"), "产品位"=w355, "槽点位"=w337, "产品位指向角度"=w345, "产品底线半径"=w364, "向外延伸距离"=w363, "向内延伸距离"=w362, "排除间隔"=w361) -> (w358:T21)
    n117 = call "cam0-制作槽边选框ROI-2.vi"("槽形状参数配置"="槽形状参数配置-槽边白条", "产品位指向角度"=w345, "槽宽"=w336, "槽点位"=w337, "Cut基点"=w338) -> ("ROI槽区"=w333:T3, "ROI槽边白条区域"=w342:T3)  [unwired: 5 in]
    n118 = Insert Into Array(array=w344, new element=w342) -> (w343:T3[])  [unwired: 1 in]
    n119 = call "cam0-镜像槽点对应中心槽角计算.vi"("位置参数"=w356) -> ("匹配到的槽角序号"=w346:i32, "槽点偏距与产品半径比"=w351:dbl)  [unwired: 8 in, 1 out]
    n120 = Insert Into Array(array=w335, new element=w333) -> (w334:T3[])  [unwired: 1 in]
    n121 = Less?(x=w351, y=w350) -> (x < y?=w328:bool)
    n122 = case shown="真" w328 {
      tunnel: [w367 w368] -> w360
      tunnel: w349 -> [_ w387]
      tunnel: w359 -> [w367 w369]
      tunnel: w336 -> [_ w383]
      tunnel: w337 -> [_ w372]
      tunnel: w355 -> [_ w373]
      tunnel: w354 -> [_ w375]
      tunnel: w345 -> [_ w374]
      tunnel: w346 -> [_ w370]
      frame False {
      }
      frame True {
        # "添加合并同一槽的不同镜像测量结果\n此处仅收集结果，控件外分类合并"
        n123 = Index Array(array=w375, index=w370) -> (element=w380:dbl)
        n124 = Subtract(x=w380, y=w374) -> (x-y=w376:dbl)
        n125 = Less Than 0?(x=w376) -> (x < 0?=w379:bool)
        n126 = Add(x=sgl 360.0, y=w376) -> (x+y=w377:dbl)
        n127 = Select(t=w377, s=w379, f=w376) -> (s? t:f=w371:dbl)
        n128 = expression code="(x/180.0)*pi" ("degrees to radians")(w371) -> (w388:dbl)
        n129 = Cosine(x=w388) -> (cos(x)=w385:dbl)
        n130 = Divide(x=w383, y=w385) -> (x/y=w382:dbl)
        n131 = Absolute Value(x=w382) -> (abs(x)=w381:dbl)
        n132 = Bundle By Name(cluster=T22 {"槽点位置"={"X"=0.0, "Y"=0.0}, "影像序号"=0, "影像位置"={"X"=0.0, "Y"=0.0}, "对应槽位序号"=0, "槽宽测量值"=0.0, "槽宽修正值"=0.0, "槽视角"=0.0} ("槽点检出信息"), "槽视角"=w371, "影像位置"=w373, "影像序号"=w387, "槽点位置"=w372, "对应槽位序号"=w370, "槽宽测量值"=w383, "槽宽修正值"=w381) -> (w384:T22)
        n133 = Insert Into Array "数组插入"(array=w369, new element=w384) -> (w368:T14)  [unwired: 1 in]
      }
    }
    n134 = case "条件结构" shown="真" FALSE {
      tunnel: w358 -> [_ w412]
      tunnel: w338 -> [_ w409]
      tunnel: w348 -> [_ w405]
      tunnel: w347 -> [_ w400]
      tunnel: w332 -> [_ w397]
      tunnel: w331 -> [w389 w391]
      tunnel: [w389 w390] -> w330
      frame False {
      }
      frame True {
        # "仅接近正对着的情况用于分析铜碎"
        n135 = Unbundle(w400) -> ("New Image"=w396:T2, "New Image"=w395:T2, "New Image"=w394:T2, "New Image"=w393:T2, "New Image"=w392:T2)
        n136 = Bundle By Name(cluster=T23 {"ImageCut"=refnum, "ImageCutGray"=refnum, "ImageMask"=refnum, "ImageInter1"=refnum, "ImageInter2"=refnum, "ImageInter3"=refnum} ("images"), "ImageCut"=w397, "ImageCutGray"=w396, "ImageMask"=w395, "ImageInter1"=w394, "ImageInter2"=w393, "ImageInter3"=w392) -> (w398:T23)
        n137 = Array Size(array=w391) -> (size(s)=w404:i32)
        n138 = Array Size(array=w405) -> (size(s)=w406:i32)
        n139 = Increment(x=w404) -> (x+1=w407:i32)
        n140 = call "cam0#-搜索铜碎-2.vi"("Cut基点"=w409, "输入参数信息"=w412, "images"=w398) -> ("检出点"=w410:cluster{"X":sgl, "Y":sgl}[], "ImageMorphOut"=w408:T2)  [unwired: 6 in, 1 out]
        n141 = Less Or Equal?(x=w407, y=w406) -> (x <= y?=w403:bool)
        n142 = And(x=w403, y="开启铜碎调试显示") -> (x .and. y?=w402:bool)
        n143 = Bundle("检出点"=w410) -> (w411:cluster{"检出点":cluster{"X":sgl, "Y":sgl}[]})  [unwired: 1 in]
        n144 = case shown="真" w402 {
          tunnel: w408 -> [_ w418]
          tunnel: w405 -> [_ w417]
          tunnel: w404 -> [_ w416]
          frame False {
          }
          frame True {
            # "直观效果调试输出"
            n145 = Index Array(array=w417, index=w416) -> (element=w415:T2)
            n146 = call "IMAQ Copy"("Image Dst"=w415, "Image Src"=w418) -> ("error out"=w413:errorcluster, "Image Dst Out"=→"Image Dst Out":T2)  [unwired: 4 in]
            n147 = call <vilib>:"Clear Errors.vi"("error in (no error)"=w413) -> ()  [unwired: 5 in, 2 out]
          }
        }
        n148 = Insert Into Array "数组插入"(array=w391, new element=w411) -> (w390:cluster{"铜碎点":cluster{"X":sgl, "Y":sgl}[]}[])  [unwired: 1 in]
      }
    }
  }
  n149 = call "IMAQ Mask"("error in (no error)"=w209, "Image Mask"=w106, "Image Src"=w229) -> ("error out"=w99:errorcluster, "Image Dst Out"=w217:T2)  [unwired: 2 in]
  n150 = call "HXQ-钩外多胶-检测.vi"("裁切偏移"=w16, "ImgRef"=w25, "MirroredAngle"=w37, "Global Rectangle"=w7, "ImageSRC"=w36) -> ("顶洞缺胶状态正常"=w4:bool, "多胶异常RECT"=w6:cluster{dbl, dbl, dbl, dbl}, "钩外多胶正常"=w35:bool)  [unwired: 3 in, 1 out]
  "钩外多胶正常" <- w35
  n151 = disable-structure shown="启用" {
    disable-tunnel: "头部缺损最大偏差" -> [w424 _]
    disable-tunnel: w163 -> [w423 _]
    disable-tunnel: [w422 w425] -> w153
    disable-tunnel: [w421 cluster{"X":dbl, "Y":dbl}[] [] ("Defect Points")] -> w148
    disable-tunnel: w135 -> [w420 _]
    disable-tunnel: [w419 0.0 ("头缺量")] -> w97
    disable-tunnel: w4 -> [_ w425]
    frame Disabled {
      n152 = call "多反-头缺检测-边线检测.vi"("缺损最大偏移量"=w424, "Annulus"=w423, "IMG_IN"=w420) -> ("Defect Points"=w421:cluster{"X":dbl, "Y":dbl}[], "Pass Status"=w422:bool, "最大值"=w419:dbl)  [unwired: 5 in, 1 out]
    }
    frame Enabled {
      (unwired) TRUE ("Pass Status")
    }
  }
  "头缺量" <- w97
  n153 = call "IMAQ Copy"("error in (no error)"=w264, "Image Dst"=w143, "Image Src"=w36) -> ("error out"=w212:errorcluster, "Image Dst Out"=w273:T2)  [unwired: 3 in]
  n154 = call <vilib>:"Clear Errors.vi"("error in (no error)"=w99) -> ()  [unwired: 5 in, 2 out]
  n155 = call "IMAQ Mask"("error in (no error)"=w212, "Image Dst"=w105, "Image Mask"=w215, "Image Src"=w211) -> ("error out"=w293:errorcluster, "Image Dst Out"=w210:T2)  [unwired: 1 in]
  n156 = Subtract(x=w192, y=w203) -> (x-y=w202:cluster{sgl, sgl})
  n157 = Merge Errors(w293, w116) -> (w274:errorcluster)
  n158 = Unbundle(w202) -> (w201:sgl, w200:sgl)
  n159 = Subtract(x=w200, y=w187) -> (x-y=w207:dbl)
  n160 = Add(x=w200, y=w187) -> (x+y=w205:dbl)
  n161 = Subtract(x=w201, y=w188) -> (x-y=w208:dbl)
  n162 = Add(x=w201, y=w188) -> (x+y=w206:dbl)
  n163 = Bundle(w208, w207, w206, w205, "MirroredAngle"=w37) -> (w204:cluster{dbl, dbl, dbl, dbl, "MirroredAngle":dbl})  [unwired: 1 in]
  n164 = disable-structure shown="启用" {
    disable-tunnel: w274 -> [w451 w453]
    disable-tunnel: w273 -> [w449 _]
    disable-tunnel: w271 -> [w448 _]
    disable-tunnel: w270 -> [w447 _]
    disable-tunnel: w257 -> [w438 _]
    disable-tunnel: w211 -> [w435 _]
    disable-tunnel: w185 -> [w433 _]
    disable-tunnel: [w432 T24 {"Left"=0, "Top"=0, "Right"=0, "Bottom"=0} ("矩形框")] -> w152
    disable-tunnel: [w431 w453] -> w127
    disable-tunnel: w104 -> [w430 _]
    frame Disabled {
      n165 = call "IMAQ SetOffset"("error in (no error)"=w451, "Y Offset"=w448, "X Offset"=w447, "Image"=w435) -> ("error out"=w450:errorcluster, "Image Out"=w442:T2)
      n166 = call "IMAQ Mask"("error in (no error)"=w450, "Image Dst"=w430, "Image Mask"=w442, "Image Src"=w449) -> ("error out"=w445:errorcluster, "Image Dst Out"=w441:T2)  [unwired: 1 in]
      n167 = call "IMAQ SetOffset"("error in (no error)"=w445, "Y Offset"=0, "X Offset"=0 ("Y Offset"), "Image"=w442) -> ("error out"=w446:errorcluster, "Image Out"=w437:T2)
      n168 = call "IMAQ Mask"("error in (no error)"=w446, "Image Mask"=w437, "Image Src"=w441) -> ("error out"=w436:errorcluster, "Image Dst Out"=w440:T2)  [unwired: 2 in]
      n169 = call "c0-胶木铜碎"("Image In"=w440, "Blue or Luma or Val or Inten Range (Color Threshold 1)"="调整下限消除头部黑区稍亮部位误判作铜碎情况", "error in"=w436) -> ("Image Out"=w429:T2, "Particle Measurements (Pixels) (Particle Analysis 1)"=w439:dbl[][], "error out"=w428:errorcluster)  [unwired: 22 in]
      n170 = call "IMAQ Dispose"("Image"=w429, "error in (no error)"=w428) -> ("error out"=w431:errorcluster)  [unwired: 4 in]
      n171 = call "cam0-输出颗粒信息.vi"("截图左上Y"=w438, "截图左上X"=w433, "颗粒分析结果"=w439) -> ("矩形框"=w432:T24)  [unwired: 6 in, 2 out]
    }
    frame Enabled {
    }
  }
  n172 = call "IMAQ Convert Rectangle to ROI"("Rectangle"=w204) -> ("ROI Descriptor"=w199:T3)  [unwired: 8 in, 1 out]
  n173 = Empty Array?(array=w222) -> (empty?=w221:bool)
  n174 = case shown="假" w221 {
    tunnel: w222 -> [w475 _]
    tunnel: w106 -> [w474 w476]
    tunnel: w210 -> [w471 w478]
    tunnel: [w456 errorcluster {"status"=FALSE, "code"=0, "source"=""} ("error out")] -> w195
    tunnel: w217 -> [w469 _]
    tunnel: [w455 w478] -> w194
    tunnel: [w463 w476] -> w198
    tunnel: w160 -> [w466 _]
    frame False {
      # "添加槽边区域以便检测槽边白条"
      n175 = call "IMAQ Group ROIs"("ROI Descriptors"=w475) -> ("error out"=w473:errorcluster, "ROI Descriptor out"=w472:T3)  [unwired: 3 in]
      n176 = call "IMAQ ROIToMask 2"("Image Model"=w471, "error in (no error)"=w473, "ROI Descriptor"=w472, "Image"=w474) -> ("error out"=w468:errorcluster, "Image Out"=w463:T2)  [unwired: 5 in, 1 out]
      n177 = call "IMAQ Or"("error in (no error)"=w468, "Image Src B"=w463, "Image Src A"=w471) -> ("error out"=w467:errorcluster, "Image Dst Out"=w470:T2)  [unwired: 7 in]
      n178 = call "IMAQ Mask"("error in (no error)"=w467, "Image Mask"=w469, "Image Src"=w470) -> ("error out"=w462:errorcluster, "Image Dst Out"=w459:T2)  [unwired: 2 in]
      n179 = call "IMAQ Group ROIs"("error in (no error)"=w462, "ROI Descriptors"=w466) -> ("error out"=w464:errorcluster, "ROI Descriptor out"=w465:T3)  [unwired: 2 in]
      n180 = call "IMAQ ROIToMask 2"("Background Value (0)"=255, "Image Model"=w459, "error in (no error)"=w464, "Filling Value (255)"=0, "ROI Descriptor"=w465, "Image"=w463) -> ("error out"=w457:errorcluster, "Image Out"=w458:T2)  [unwired: 3 in, 1 out]
      n181 = call "IMAQ And"("error in (no error)"=w457, "Image Src B"=w458, "Image Src A"=w459) -> ("error out"=w456:errorcluster, "Image Dst Out"=w455:T2)  [unwired: 7 in]
      n182 = Wait (ms) "均衡负载"(milliseconds to wait=u32 3 ("等待时间（毫秒）")) -> ()  [unwired: 1 out]
    }
    frame True {
    }
  }
  n183 = disable-structure shown="启用" {
    frame Disabled {
      n184 = local read "镜像编号"() -> ()  [unwired: 1 out]
    }
    frame Enabled {
    }
  }
  n185 = call "IMAQ ROIToMask 2"("Image Model"=w194, "error in (no error)"=w195, "ROI Descriptor"=w199, "Image"=w198) -> ("error out"=w196:errorcluster, "Image Out"=w197:T2)  [unwired: 5 in, 1 out]
  n186 = flat-sequence {
    tunnel: w115 -> [w481]
    tunnel: [w480] -> w123
    tunnel: [w479] -> w116
    tunnel: w117 -> [w479]
    frame #0 {
      n187 = Tick Count (ms)() -> (millisecond timer value=w482:u32)
      n188 = Subtract(x=w482, y=w481) -> (x-y=w480:u32)
    }
  }
  n189 = call "IMAQ And"("error in (no error)"=w196, "Image Src B"=w197, "Image Src A"=w194) -> ("error out"=w117:errorcluster, "Image Dst Out"=w46:T2)  [unwired: 7 in]
  "Image 3" <- w46
  n190 = call "IMAQ Mask"("Image Dst"=w144, "Image Mask"=w46, "Image Src"=w36) -> ("error out"=w102:errorcluster, "Image Dst Out"=w100:T2)  [unwired: 2 in]
  n191 = disable-structure shown="启用" {
    disable-tunnel: w103 -> [w501 _]
    disable-tunnel: w102 -> [w500 w502]
    disable-tunnel: [w494 w502] -> w101
    disable-tunnel: w46 -> [w491 _]
    disable-tunnel: w100 -> [w488 _]
    disable-tunnel: [w483 0.0] -> _
    frame Disabled {
      w495 = 0 items=["Red", "Green", "Blue", "Hue", "Saturation", "Luminance", "Value", "Intensity"] ("Color Plane")
      w496 = u32 1 items=["Bright Objects", "Dark Objects"] ("Look For (Bright Objects)")
      w499 = u32 1 items=["Niblack", "Background Correction"] ("Method")
      n192 = call "IMAQ ExtractSingleColorPlane"("Color Plane"=w495, "error in (no error)"=w500, "Image Dst"=w501, "Image Src"=w488) -> ("error out"=w494:errorcluster, "Image Dst Out"=w493:T2)  [unwired: 6 in]
      n193 = call "IMAQ Local Threshold"("Image Src"=w493, "Look For (Bright Objects)"=w496, "Method (Niblack)"=w499, "Window Size (32x32)"=cluster{"SizeX":i32, "SizeY":i32} {"SizeX"=16, "SizeY"=16} ("Kernel Size"), "error in (no error)"=w494, "Niblack/Sauvola Deviation Factor (0.2)"=0.2 ("Niblack Deviation Factor"), "Replace Value (1)"=sgl 255.0) -> ("Image Dst Out"=w487:T2, "error out"=w492:errorcluster)  [unwired: 2 in, 5 out]
      n194 = call "IMAQ And"("error in (no error)"=w492, "Image Src B"=w491, "Image Src A"=w487) -> ("error out"=w489:errorcluster, "Image Dst Out"=w486:T2)  [unwired: 7 in]
      n195 = call "c0-压点伤"("Image In"=w486, "error in"=w489) -> ("Particle Measurements (Pixels) (Particle Analysis 1)"=w484:dbl[][], "error out"=w485:errorcluster)  [unwired: 23 in, 1 out]
      n196 = call <vilib>:"Clear Errors.vi"("error in (no error)"=w485) -> ()  [unwired: 5 in, 2 out]
      n197 = Array Max & Min(array=w484) -> (max value=w483:dbl)  [unwired: 3 out]
    }
    frame Enabled {
    }
  }
  n198 = call "IMAQ ExtractSingleColorPlane"("Color Plane"=w292, "error in (no error)"=w101, "Image Dst"=w138, "Image Src"=w100) -> ("error out"=w291:errorcluster, "Image Dst Out"=w89:T2)  [unwired: 6 in]
  n199 = call "IMAQ GetImageSize"("Image"=w89) -> ("Y Resolution"=w87:i32, "X Resolution"=w79:i32, "error out"=w45:errorcluster)  [unwired: 3 in]
  n200 = call "IMAQ Threshold"("Replace Value"=sgl 1.0, "error in (no error)"=w291, "Range"=cluster{"Lower value":sgl, "Upper value":sgl} {"Lower value"=10.0, "Upper value"=200.0}, "Image Dst"=w94, "Image Src"=w89) -> ("error out"=w283:errorcluster, "Image Dst Out"=w286:T2)  [unwired: 5 in]
  n201 = Multiply(x=w87, y=0.5) -> (x*y=w84:dbl)
  n202 = To Double Precision Float(number=w79) -> (double precision float=w78:dbl)
  n203 = Multiply(x=w87, y=0.25) -> (x*y=w85:dbl)
  n204 = Subtract(x=w84, y=w85) -> (x-y=w92:dbl)
  n205 = Add(x=w84, y=w85) -> (x+y=w91:dbl)
  n206 = call "IMAQ Morphology"("Number of iterations (1)"=w280, "Structuring Element"=i32[][] [[0, 0, 1, 0, 0], [0, 1, 1, 1, 0], [1, 1, 1, 1, 1], [0, 1, 1, 1, 0], [0, 0, 1, 0, 0]], "error in (no error)"=w283, "Operation"=T12."Erode", "Image Src"=w286) -> ("error out"=w282:errorcluster, "Image Dst Out"=w284:T2)  [unwired: 5 in]
  n207 = Bundle("y"=0.0, w92, w78, w91, "MirroredAngle"=w37) -> (w90:T25)  [unwired: 1 in]
  n208 = call "IMAQ SetOffset"("error in (no error)"=w282, "Y Offset"=0, "X Offset"=0, "Image"=w284) -> ("error out"=w256:errorcluster, "Image Out"=w75:T2)
  n209 = call "IMAQ Convert Rectangle to ROI"("error in (no error)"=w45, "Rectangle"=w90) -> ("error out"=w44:errorcluster, "ROI Descriptor"=w72:T3)  [unwired: 7 in]
  n210 = call "IMAQ Mask"("error in (no error)"=w44, "Image Mask"=w75, "Image Src"=w89) -> ("error out"=w58:errorcluster, "Image Dst Out"=w73:T2)  [unwired: 2 in]
  n211 = disable-structure shown="禁用" {
    disable-tunnel: w256 -> [w511 w512]
    disable-tunnel: [w509 w512] -> w255
    disable-tunnel: [w508 _] -> w193
    disable-tunnel: w100 -> [w507 _]
    disable-tunnel: w93 -> [w506 _]
    disable-tunnel: w75 -> [w505 _]
    disable-tunnel: [w504 _] -> w62
    frame Disabled {
      n212 = call "IMAQ Mask"("error in (no error)"=w511, "Image Mask"=w505, "Image Src"=w507) -> ("error out"=w510:errorcluster, "Image Dst Out"=w504:T2)  [unwired: 2 in]
      n213 = call "c0-白条"("Image In"=w504, "Image Dst"=w506, "error in"=w510) -> ("Particle Measurements (Pixels) (Parts_Zn)"=w508:dbl[][], "error out"=w509:errorcluster)  [unwired: 22 in, 1 out]
    }
    frame Enabled {
    }
  }
  n214 = call "IMAQ Overlay ROI"("ROI Descriptor"=w72, "Image"=w73) -> ("error out"=w43:errorcluster, "Image Out"=w5:T2)  [unwired: 8 in]
  "脏污检测图像" <- w5
  n215 = call <vilib>:"Clear Errors.vi"("error in (no error)"=w43) -> ()  [unwired: 5 in, 2 out]
  n216 = call "IMAQ Morphology"("Number of iterations (1)"=3, "error in (no error)"=w58, "Operation"=T12."Erode", "Image Src"=w75) -> ("error out"=w57:errorcluster, "Image Dst Out"=w69:T2)  [unwired: 6 in]
  n217 = call "IMAQ Multiply"("Image Src A"=w69, "Constant"=250.0, "error in (no error)"=w57) -> ("Image Dst Out"=w63:T2, "error out"=w56:errorcluster)  [unwired: 4 in]
  n218 = call "IMAQ Rake 3"("Image"=w5, "Edge Options"="检刀纹_EdgeOptions", "Optimized Mode"=FALSE, "ROI Descriptor"=w72, "Step Size"=u32 7, "Process"=T13."Get All Edges") -> ("Search Lines"=w71:T26[])  [unwired: 6 in, 3 out]
  n219 = call <vilib>:"Clear Errors.vi"("error in (no error)"=w56) -> ()  [unwired: 5 in, 2 out]
  n220 = call "Vision Assistant"("Image In"=w5, "Range (Threshold 1)"="脏污灰度上限", "Selection Values (Particle Filter 1)"="脏污面积下限") -> ("Number of Particles (Particle Analysis 1)"=w39:i32, "Particle Measurements (Pixels) (Particle Analysis 1)"=→"脏污所处位置信息":dbl[][])  [unwired: 21 in, 2 out]
  "脏污数量" <- w39
  n221 = for {
    tunnel: w71 -> [w518] mode=indexing
    shift-right: [w515] -> w66
    shift-left: w63 -> [w516]
    shift-right: [w513] -> w64
    shift-left: cluster{"X":sgl, "Y":sgl}[] [] -> [w514]
    n222 = Unbundle By Name(w518) -> ("Edge Info"=w517:T18[])
    n223 = for {
      tunnel: w517 -> [w527] mode=indexing
      shift-right: [w528] -> w515
      shift-left: w516 -> [w526]
      shift-right: [w520] -> w513
      shift-left: w514 -> [w521]
      n224 = Unbundle By Name(w527) -> ("Location (Pixel)"=w519:cluster{"X":sgl, "Y":sgl})
      n225 = Unbundle(w519) -> ("X"=w525:sgl, "Y"=w524:sgl)
      n226 = call "IMAQ GetPixelValue"("Image"=w526, "X Coordinate"=w525, "Y Coordinate"=w524) -> ("Pixel Value (U8)"=w523:u8)  [unwired: 3 in, 4 out]
      n227 = Greater Than 0?(x=w523) -> (x > 0?=w522:bool)
      n228 = case shown="真" w522 {
        tunnel: w521 -> [w530 w533]
        tunnel: [w530 w532] -> w520
        tunnel: w519 -> [_ w531]
        frame False {
        }
        frame True {
          n229 = Insert Into Array(array=w533, new element=w531) -> (w532:cluster{"X":sgl, "Y":sgl}[])  [unwired: 1 in]
        }
      }
      n230 = call "IMAQ Overlay Points"("Color"=u32 6618880, "Point"=w519, "Image"=w526) -> ("Image Out"=w528:T2)  [unwired: 7 in, 1 out]
    }
  }
  n231 = disable-structure shown="启用" {
    disable-tunnel: w62 -> [w537 _]
    disable-tunnel: w1 -> [w535 _]
    frame Disabled {
      n232 = Not(x=w535) -> (.not. x?=w534:bool)
      n233 = call "img1log.vi"("使能"=w534, "相机名称"="cam0——白条", "srcImage"=w537) -> ()  [unwired: 7 in, 2 out]
    }
    frame Enabled {
    }
  }
  n234 = call "cam0-输出颗粒信息.vi"("截图左上Y"=w257, "截图左上X"=w185, "白条面积限度"="白条面积限度", "颗粒分析结果"=w193) -> ("矩形框"=w122:T24)  [unwired: 5 in, 2 out]
  n235 = Greater Than 0?(x=w39) -> (x > 0?=w61:bool)
  n236 = call "IMAQ Overlay Points"("Color"=u32 16711680, "Array of Points"=w64, "Image"=w66) -> ("error out"=w42:errorcluster, "Image Out"=→"用于打探针查看":T2)  [unwired: 7 in]
  n237 = Empty Array?(array=w64) -> ()  [unwired: 1 out]
  n238 = call <vilib>:"Clear Errors.vi"("error in (no error)"=w42) -> ()  [unwired: 5 in, 2 out]
  n239 = Merge Errors(w255, w127) -> (→"错误输出":errorcluster)
  n240 = Bundle By Name(cluster=T4 {"HeadOK"=FALSE, "白条检出位置"={"Left"=0, "Top"=0, "Right"=0, "Bottom"=0}, "胶木铜碎检出位置"={"Left"=0, "Top"=0, "Right"=0, "Bottom"=0}, "白条ok"=FALSE, "ROI头缺检测显示"={"Global Rectangle"=[], "Contours"=[]}, "头缺检出位置"=[], "槽检测信息"=[], "铜碎信息每元素一条槽"=[{"铜碎点"=[]}, {"铜碎点"=[]}, {"铜碎点"=[]}, {"铜碎点"=[]}, {"铜碎点"=[{"X"=0.0, "Y"=0.0}]}], "点伤"=0.0, "脏污"=FALSE, "钩外多胶"=FALSE, "多胶异常RECT"={0.0, 0.0, 0.0, 0.0}}, "HeadOK"=w153, "白条检出位置"=w122, "胶木铜碎检出位置"=w152, "白条ok"=w1, "ROI头缺检测显示"=w149, "头缺检出位置"=w148, "槽检测信息"=w146, "铜碎信息每元素一条槽"=w60, "点伤"=w97, "脏污"=w61, "钩外多胶"=w35, "多胶异常RECT"=w6) -> (→"输出簇":T4)
  n241 = Bundle(w114, w124, w123) -> (→"ms":cluster{u32, u32, u32})  [unwired: 1 in]
